vi "SaveDeviceHeader.vi"(0 "File Refnum in":refnum<file>, 1 "no. of arrays":i32, 3 "Array Lengths":i32, 5 "Filename":string, 7 "Run Number":i32, 9 "Array Titles":string, 11 "error in (no error)":errorcluster, 12 "Temperature":dbl, 13 "Humidity":dbl, 14 "Strip Segment":string) -> (4 "File Refnum out":refnum<file>, 6 "Header string":string, 10 "error out":errorcluster)   [LabVIEW 2018]
uses:
  globals/QC_RunInformation.vi
  globals/QC_MeasurementSetup.vi
  <vilib>/regexp/Match Regular Expression.xnode
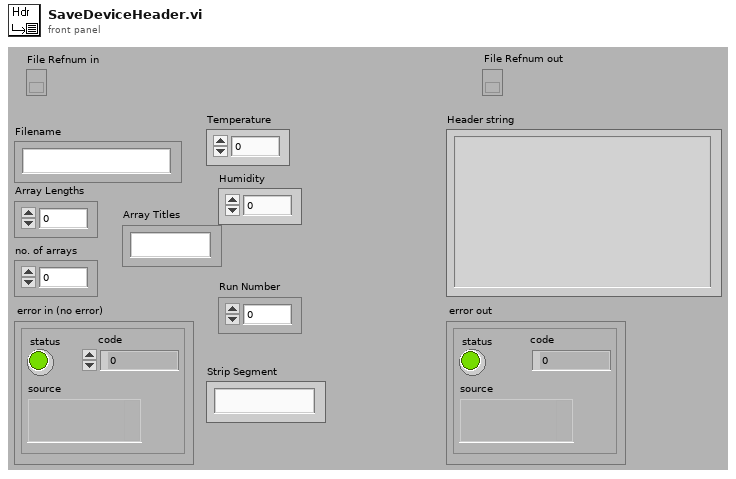
[diagram p1: front panel]
types:
  T1 = cluster{"Institute":string, "Manufacturers":string[], "Devices":string[], "Serialnumbers Lookup DB":string, "Data directory":string, "Backup & screenshot directory":string, "List of known users":string[], "Measurement switch not used":bool, "Measurement Switch":string, "DUT Switch":string, "Rseries IV [MOhm]":string, "Rshunt IV [MOhm]":string, "Rseries CV [MOhm]":string, "DC blocking Cap [µF]":string, "Rseries LCR [MOhm]":string, "Rseries stability [MOhm]":string, "Rshunt stability [MOhm]":string, "Rseries striptest bias [MOhm]":string, "Rseries strip pinhole [MOhm]":string}
  T2 = cluster{"Sensor Serial No.:":string, "Wafer:":string, "Batch:":string, "Manufacturer:":string, "Device Category:":string, "Database Serial No.:":string, "Date Initiated:":string, "Time Initiated:":string, "Test":string, "Probeplan used:":string, "End of Run comment:":string, "User:":string, "Vbias SMU":string, "LCR":string, "Test SMU":string, "Test DMM":string}
  T3 = cluster{"Supply":refnum<class "SupplyControl.lvclass">, "LCR":refnum<class "LCRControl.lvclass">, "Arduino":refnum<class "ArduinoControl.lvclass">, "Measurement switch":refnum<class "Switching.lvclass">, "Initial Voltage [V]":dbl, "Final Voltage [V]":dbl, "Step Size [V]":dbl, "Step Interval [s]":i32, "Number Of Steps":u32, "AC frequency [Hz]":i32, "RC Configuration":u16, "AC amplitude [V]":dbl, "Ramp down steps [V]":dbl, "Ramp down Interval [s]":i32, "Set Current Limit?":bool, "Current Limit [µA]":dbl, "Temperature Readout":enum16{"Read Arduino", "Enter manually"}, "Supply Name":string, "LCR Name":string, "V_depletion Limit [V]":dbl, "Measurement switch used?":bool}
  T4 = cluster{"Bias Supply":refnum<class "SupplyControl.lvclass">, "SMU":refnum<class "SupplyControl.lvclass">, "LCR":refnum<class "LCRControl.lvclass">, "ProbeStation":refnum<class "ProbeStationControl.lvclass">, "Arduino":refnum<class "ArduinoControl.lvclass">, "Measurement switch":refnum<class "Switching.lvclass">, "Probe Card Channels":i32, "Bias Voltage [V]":dbl, "First strip":i32, "Last strip":i32, "Base Voltage [V]":dbl, "Base Ramp Step [V]":dbl, "Base Ramp Interval [ms]":u32, "High Voltage [V]":dbl, "High Ramp Step [V]":dbl, "High Ramp Interval [ms]":u32, "AC frequency [Hz]":i32, "AC amplitude [V]":dbl, "RC Configuration":u16, "Single Needle":bool, "Temperature Readout":enum16{"Read Arduino", "Enter manually"}, "Fraction of good strips [%]":dbl, "Measurement switch used?":bool, "Matrix X Channels":cluster{"Mux1 C1":i32, "Mux1 C2":i32, "Mux2 C1":i32, "Mux2 C2":i32}, "Pinholes Y/N":bool, "Capacitance Y/N":bool, "Resistance Y/N":bool, "Bias Supply Name":string, "SMU Name":string, "LCR Name":string}
  T5 = cluster{"Supply":refnum<class "SupplyControl.lvclass">, "LCR":refnum<class "LCRControl.lvclass">, "Arduino":refnum<class "ArduinoControl.lvclass">, "Measurement switch":refnum<class "Switching.lvclass">, "Initial Voltage [V]":dbl, "Final Voltage [V]":dbl, "Step Size [V]":dbl, "Step Interval [s]":i32, "Number Of Steps":u32, "AC frequency [Hz]":i32, "RC Configuration":u16, "AC amplitude [V]":dbl, "Ramp down steps [V]":dbl, "Ramp down Interval [s]":i32, "Set Current Limit?":bool, "Current Limit [µA]":dbl, "Temperature Readout":enum16{"Read Arduino", "Enter manually"}, "Supply Name":string, "LCR Name":string, "C_is Limit [pF/cm]":dbl, "Measurement switch used?":bool}
  T6 = cluster{"Bias Supply":refnum<class "SupplyControl.lvclass">, "SMU":refnum<class "SupplyControl.lvclass">, "Arduino":refnum<class "ArduinoControl.lvclass">, "Initial Voltage [V]":dbl, "Final Voltage [V]":dbl, "Step Size [V]":dbl, "Step Interval [s]":i32, "Number Of Steps":u32, "Ramp down steps [V]":dbl, "Ramp down Interval [s]":i32, "Bias Voltage [V]":dbl, "Set Current Limit?":bool, "Current Limit [µA]":dbl, "Temperature Readout":enum16{"Read Arduino", "Enter manually"}, "Bias Supply Name":string, "SMU Name":string}
  T7 = cluster{"Supply":refnum<class "SupplyControl.lvclass">, "DMM":refnum<class "MultimeterControl.lvclass">, "DUT switch":refnum<class "Switching.lvclass">, "Arduino":refnum<class "ArduinoControl.lvclass">, "Measurement switch":refnum<class "Switching.lvclass">, "Voltage [V]":dbl, "Measurement Interval [s]":i32, "Test Duration":u32, "Ramp up steps [V]":dbl, "Ramp up Interval [s]":u32, "Ramp down steps [V]":dbl, "Ramp down Interval [s]":i32, "Set Current Limit?":bool, "Current Limit [µA]":dbl, "Temperature Readout":enum16{"Read Arduino", "Enter manually"}, "Supply Name":string, "DMM Name":string, "Maximum current fluctuation [%]":dbl, "Measurement switch used?":bool, "DUT switch used?":bool}
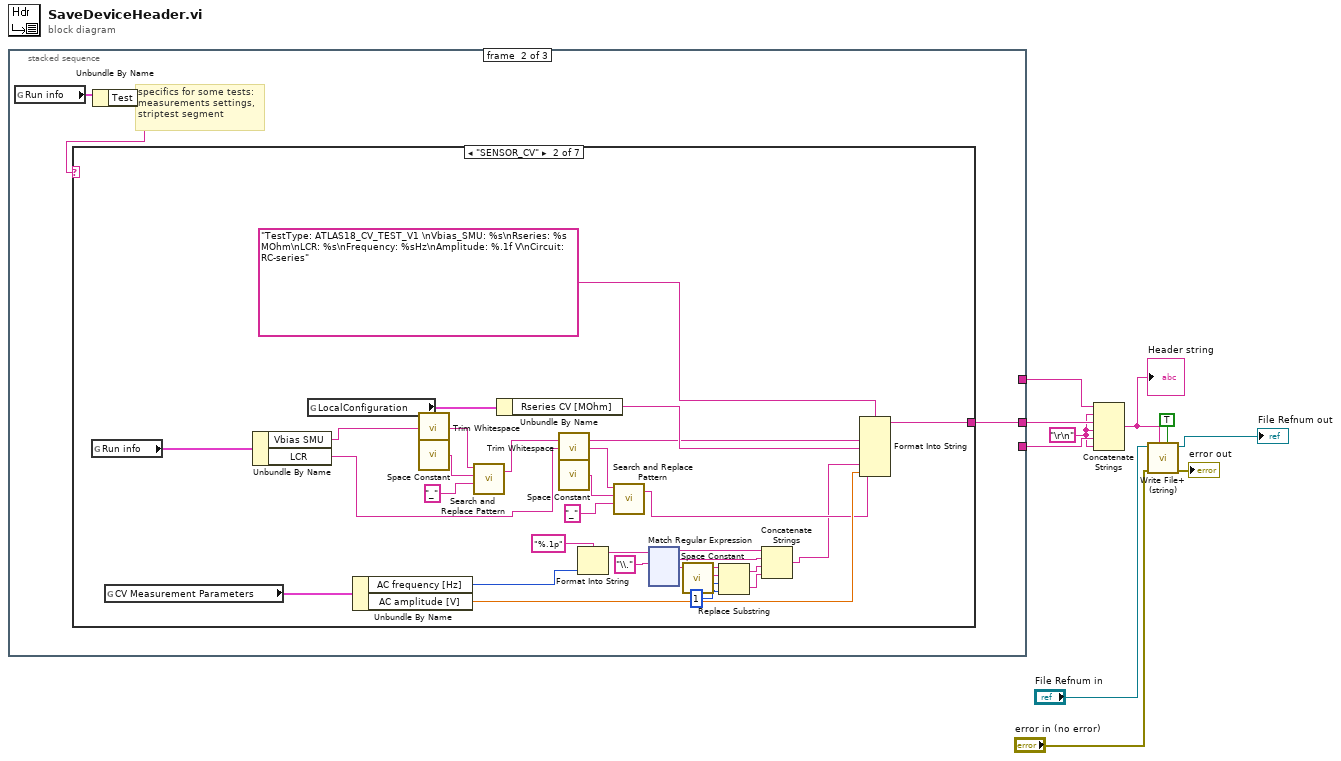
[diagram p0: block diagram]
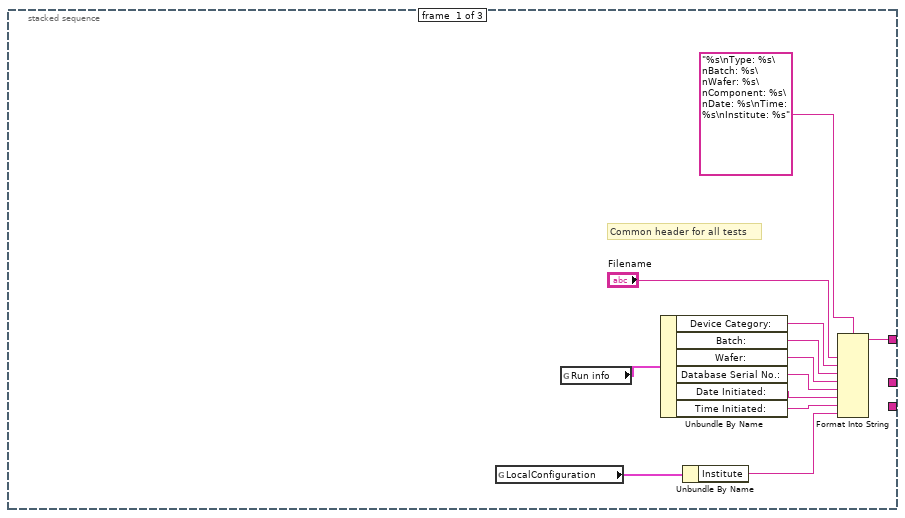
[diagram p2: hidden frame]
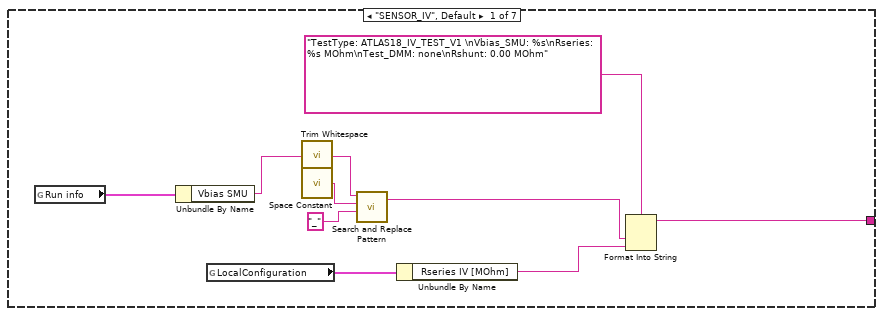
[diagram p3: hidden frame]
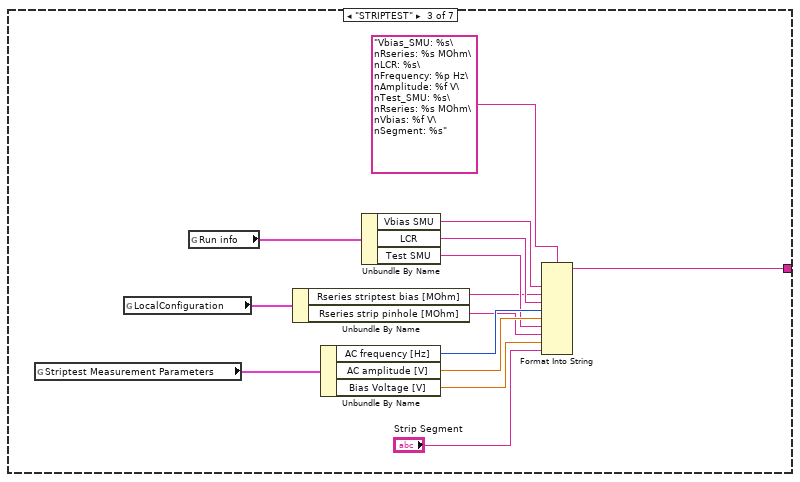
[diagram p4: hidden frame]
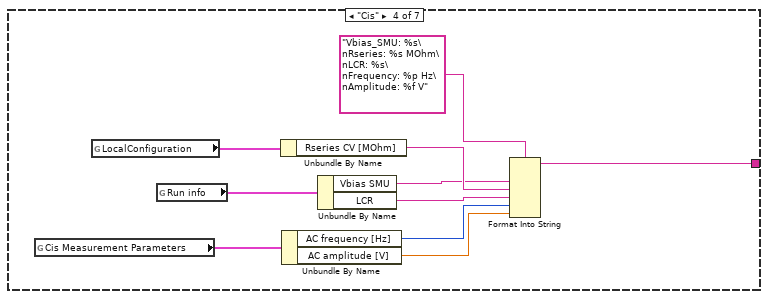
[diagram p5: hidden frame]
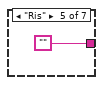
[diagram p6: hidden frame]
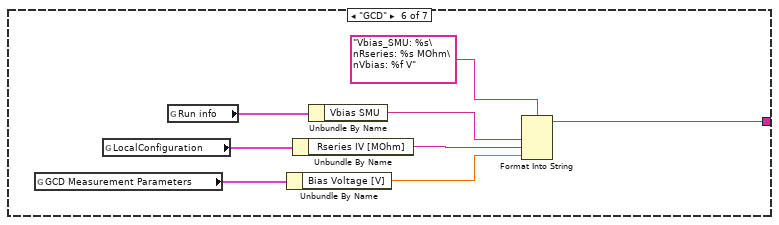
[diagram p7: hidden frame]
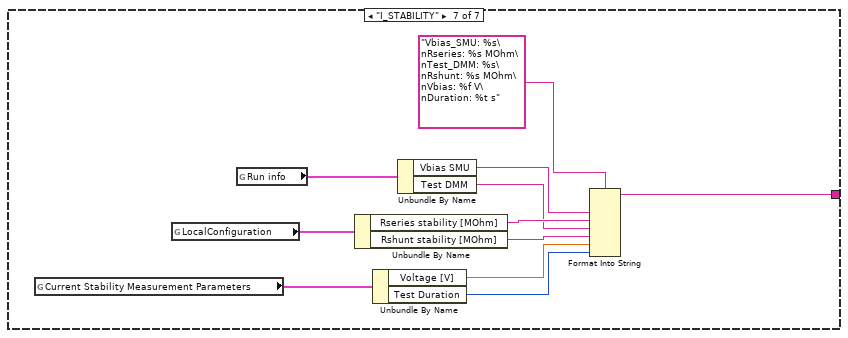
[diagram p8: hidden frame]
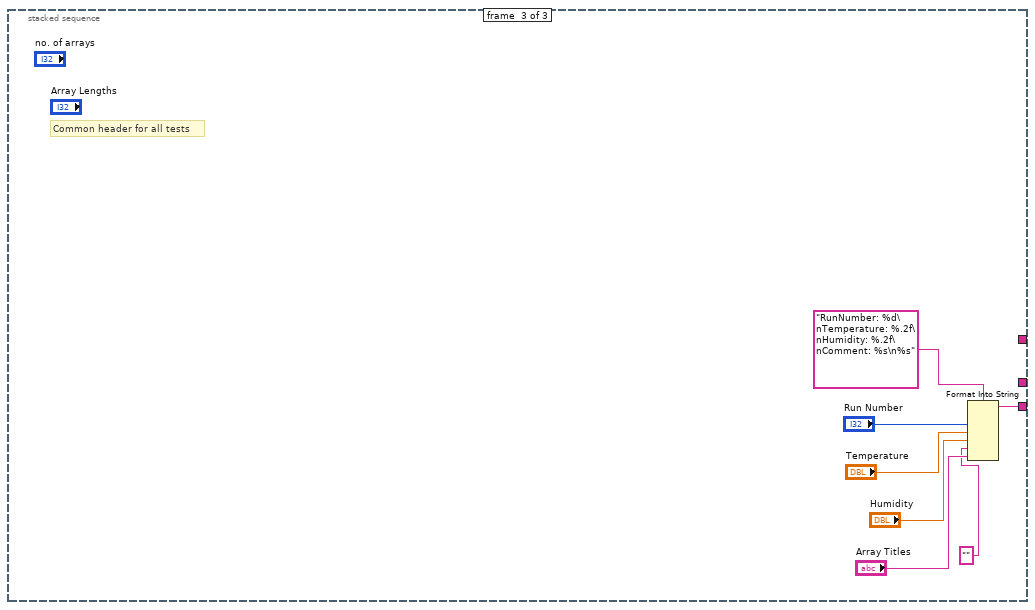
[diagram p9: hidden frame]
diagram:
  w2 = "\r\n"
  n1 = stacked-sequence {
    tunnel: [_ w25 _] -> w6
    tunnel: [_ _ w225] -> w5
    tunnel: [w11 _ _] -> w4
    frame #0 {
      # "Common header for all tests"
      n2 = global read "QC_RunInformation.vi" "LocalConfiguration"() -> (w12:T1)
      n3 = global read "QC_RunInformation.vi" "Run info"() -> (w13:T2)
      n4 = Unbundle By Name(w13) -> ("Device Category:"=w16:string, "Batch:"=w17:string, "Wafer:"=w18:string, "Database Serial No.:"=w19:string, "Date Initiated:"=w20:string, "Time Initiated:"=w21:string)
      n5 = Unbundle By Name(w12) -> ("Institute"=w22:string)
      n6 = Format Into String(format string="%s\nType: %s\nBatch: %s\nWafer: %s\nComponent: %s\nDate: %s\nTime: %s\nInstitute: %s", "Filename", w16, w17, w18, w19, w20, w21, w22) -> (resulting string=w11:string)  [unwired: 2 in, 1 out]
    }
    frame #1 {
      # "specifics for some tests:\nmeasurements settings,\nstriptest segment"
      n7 = global read "QC_RunInformation.vi" "Run info"() -> (w24:T2)
      n8 = Unbundle By Name(w24) -> ("Test"=w23:string)
      n9 = case shown="\"SENSOR_CV\"" w23 {
        tunnel: [w31 w58 w189 w193 "" w204 w218] -> w25
        frame "SENSOR_IV", Default {
          n10 = global read "QC_RunInformation.vi" "Run info"() -> (w34:T2)
          n11 = Unbundle By Name(w34) -> ("Vbias SMU"=w28:string)
          n12 = global read "QC_RunInformation.vi" "LocalConfiguration"() -> (w35:T1)
          n13 = call <vilib>:"Trim Whitespace.vi"("string"=w28) -> ("trimmed string"=w27:string)  [unwired: 1 in]
          n14 = call <vilib>:"Space Constant.vi"() -> ("String"=w30:string)
          n15 = call <vilib>:"Search and Replace Pattern.vi"("string"=w27, "regular expression (\"\")"=w30, "replace string (\"\")"="_" ("replace string (\"\")")) -> ("result string"=w26:string)  [unwired: 2 in, 1 out]
          n16 = Unbundle By Name(w35) -> ("Rseries IV [MOhm]"=w32:string)
          n17 = Format Into String(format string="TestType: ATLAS18_IV_TEST_V1 \nVbias_SMU: %s\nRseries: %s MOhm\nTest_DMM: none\nRshunt: 0.00 MOhm", w26, w32) -> (resulting string=w31:string)  [unwired: 2 in, 1 out]
        }
        frame "SENSOR_CV" {
          w42 = 1 ("offset (0)")
          n18 = global read "QC_RunInformation.vi" "Run info"() -> (w62:T2)
          n19 = global read "QC_MeasurementSetup.vi" "CV Measurement Parameters"() -> (w64:T3)
          n20 = Unbundle By Name(w62) -> ("Vbias SMU"=w54:string, "LCR"=w49:string)
          n21 = global read "QC_RunInformation.vi" "LocalConfiguration"() -> (w63:T1)
          n22 = Unbundle By Name(w64) -> ("AC frequency [Hz]"=w37:i32, "AC amplitude [V]"=w59:dbl)
          n23 = call <vilib>:"Trim Whitespace.vi"("string"=w54) -> ("trimmed string"=w55:string)  [unwired: 1 in]
          n24 = call <vilib>:"Space Constant.vi"() -> ("String"=w57:string)
          n25 = call <vilib>:"Search and Replace Pattern.vi"("string"=w55, "regular expression (\"\")"=w57, "replace string (\"\")"="_" ("replace string (\"\")")) -> ("result string"=w53:string)  [unwired: 2 in, 1 out]
          n26 = Unbundle By Name(w63) -> ("Rseries CV [MOhm]"=w60:string)
          n27 = call <vilib>:"Trim Whitespace.vi"("string"=w49) -> ("trimmed string"=w50:string)  [unwired: 1 in]
          n28 = call <vilib>:"Space Constant.vi"() -> ("String"=w52:string)
          n29 = Format Into String(format string="%.1p", w37) -> (resulting string=w45:string)  [unwired: 2 in, 1 out]
          n30 = call <vilib>:"Search and Replace Pattern.vi"("string"=w50, "regular expression (\"\")"=w52, "replace string (\"\")"="_" ("replace string (\"\")")) -> ("result string"=w48:string)  [unwired: 2 in, 1 out]
          n31 = xnode "Match Regular Expression"("input string"=w45, "regular expression"="\\.") -> ("before match"=w41:string, "whole match"=w40:string, "after match"=w44:string)  [unwired: 4 in, 2 out]
          n32 = call <vilib>:"Space Constant.vi"() -> ("String"=w43:string)
          n33 = Replace Substring(2:w42, 3:w42, 4:w43, 5:w44) -> (0:w38:string, 1:w39:string)
          n34 = Concatenate Strings(w41, w40, w39, w38) -> (w36:string)
          n35 = Format Into String(format string="TestType: ATLAS18_CV_TEST_V1 \nVbias_SMU: %s\nRseries: %s MOhm\nLCR: %s\nFrequency: %sHz\nAmplitude: %.1f V\nCircuit: RC-series", w53, w60, w48, w36, w59) -> (resulting string=w58:string)  [unwired: 2 in, 1 out]
        }
        frame "STRIPTEST" {
          n36 = global read "QC_MeasurementSetup.vi" "Striptest Measurement Parameters"() -> (w191:T4)
          n37 = global read "QC_RunInformation.vi" "LocalConfiguration"() -> (w182:T1)
          n38 = global read "QC_RunInformation.vi" "Run info"() -> (w192:T2)
          n39 = Unbundle By Name(w182) -> ("Rseries striptest bias [MOhm]"=w181:string, "Rseries strip pinhole [MOhm]"=w179:string)
          n40 = Unbundle By Name(w191) -> ("AC frequency [Hz]"=w188:i32, "AC amplitude [V]"=w187:dbl, "Bias Voltage [V]"=w180:dbl)
          n41 = Unbundle By Name(w192) -> ("Vbias SMU"=w185:string, "LCR"=w184:string, "Test SMU"=w183:string)
          n42 = Format Into String(format string="Vbias_SMU: %s\nRseries: %s MOhm\nLCR: %s\nFrequency: %p Hz\nAmplitude: %f V\nTest_SMU: %s\nRseries: %s MOhm\nVbias: %f V\nSegment: %s", w185, w181, w184, w188, w187, w183, w179, w180, "Strip Segment") -> (resulting string=w189:string)  [unwired: 2 in, 1 out]
        }
        frame "Cis" {
          n43 = global read "QC_MeasurementSetup.vi" "Cis Measurement Parameters"() -> (w202:T5)
          n44 = global read "QC_RunInformation.vi" "LocalConfiguration"() -> (w201:T1)
          n45 = global read "QC_RunInformation.vi" "Run info"() -> (w200:T2)
          n46 = Unbundle By Name(w201) -> ("Rseries CV [MOhm]"=w198:string)
          n47 = Unbundle By Name(w202) -> ("AC frequency [Hz]"=w195:i32, "AC amplitude [V]"=w194:dbl)
          n48 = Unbundle By Name(w200) -> ("Vbias SMU"=w197:string, "LCR"=w196:string)
          n49 = Format Into String(format string="Vbias_SMU: %s\nRseries: %s MOhm\nLCR: %s\nFrequency: %p Hz\nAmplitude: %f V", w197, w198, w196, w195, w194) -> (resulting string=w193:string)  [unwired: 2 in, 1 out]
        }
        frame "Ris" {
        }
        frame "GCD" {
          n50 = global read "QC_MeasurementSetup.vi" "GCD Measurement Parameters"() -> (w206:T6)
          n51 = global read "QC_RunInformation.vi" "LocalConfiguration"() -> (w211:T1)
          n52 = global read "QC_RunInformation.vi" "Run info"() -> (w210:T2)
          n53 = Unbundle By Name(w206) -> ("Bias Voltage [V]"=w205:dbl)
          n54 = Unbundle By Name(w211) -> ("Rseries IV [MOhm]"=w208:string)
          n55 = Unbundle By Name(w210) -> ("Vbias SMU"=w207:string)
          n56 = Format Into String(format string="Vbias_SMU: %s\nRseries: %s MOhm\nVbias: %f V", w207, w208, w205) -> (resulting string=w204:string)  [unwired: 2 in, 1 out]
        }
        frame "I_STABILITY" {
          n57 = global read "QC_MeasurementSetup.vi" "Current Stability Measurement Parameters"() -> (w222:T7)
          n58 = global read "QC_RunInformation.vi" "LocalConfiguration"() -> (w221:T1)
          n59 = global read "QC_RunInformation.vi" "Run info"() -> (w220:T2)
          n60 = Unbundle By Name(w221) -> ("Rseries stability [MOhm]"=w216:string, "Rshunt stability [MOhm]"=w214:string)
          n61 = Unbundle By Name(w222) -> ("Voltage [V]"=w213:dbl, "Test Duration"=w212:u32)
          n62 = Unbundle By Name(w220) -> ("Vbias SMU"=w217:string, "Test DMM"=w215:string)
          n63 = Format Into String(format string="Vbias_SMU: %s\nRseries: %s MOhm\nTest_DMM: %s\nRshunt: %s MOhm\nVbias: %f V\nDuration: %t s", w217, w216, w215, w214, w213, w212) -> (resulting string=w218:string)  [unwired: 2 in, 1 out]
        }
      }
    }
    frame #2 {
      # "Common header for all tests"
      n64 = Format Into String(format string="RunNumber: %d\nTemperature: %.2f\nHumidity: %.2f\nComment: %s\n%s", "Run Number", "Temperature", "Humidity", "" ("input 5"), "Array Titles") -> (resulting string=w225:string)  [unwired: 2 in, 1 out]
    }
  }
  n65 = Concatenate Strings(w4, w2, w6, w2, w5, w2) -> (w3:string)
  "Header string" <- w3
  n66 = call <vilib>:"Write File+ (string).vi"("convert eol? (no:F)"=TRUE, "string"=w3, "error in (no error)"="error in (no error)", "refnum"="File Refnum in") -> ("error out"=→"error out":errorcluster, "dup refnum"=→"File Refnum out":refnum<file>)  [unwired: 3 in, 1 out]
